vi "Pre Launch Init.vi"(11 "VMR Actor in":refnum<class "VMR Actor.lvclass">) -> (0 "error out":errorcluster, 3 "VMR Actor out":refnum<class "VMR Actor.lvclass">)   [LabVIEW 2022 SP3, in "VMR Server.lvlib" / "VMR Actor.lvclass"]
doc: "(<B>Filename</B>: Actor Framework.lvlib:Actor.lvclass:Pre Launch Init.vi)\n\nDefines behavior that occurs after the Launch Actor method is invoked but before the actor's Actor Core method begins running.\n\nThe Pre Launch Init method is guaranteed to finish before the Launch Actor method returns to its caller and before the actor itself receives any messages. Any references that the Pre Launch Init method obtains are guaranteed to have the same lifetime as the actor itself. Any errors that the Pre Launch Init method returns will abort the launch.\n\nBy default, this method does nothing. A descendant class may override it to define behavior."
uses:
  VMR Actor.lvclass
  <vilib>/ActorFramework/Actor/Actor.lvclass
  VMR Actor.lvclass/VMR Actor.ctl
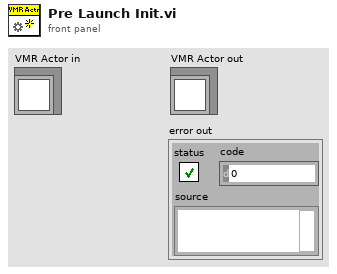
[diagram p1: front panel]
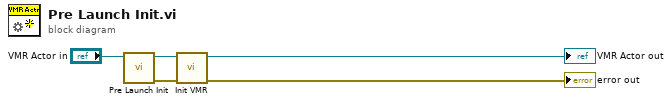
[diagram p0: block diagram]
diagram:
  n1 = call-parent "Pre Launch Init.vi"("Actor in"="VMR Actor in") -> ("error out"=w4:errorcluster, "Actor out"=w2:refnum<class "VMR Actor.lvclass">)  [unwired: 9 in]
  n2 = call "Init VMR.vi"("error in (no error)"=w4, "VMR Actor in"=w2) -> ("error out"=→"error out":errorcluster, "VMR Actor out"=→"VMR Actor out":refnum<class "VMR Actor.lvclass">)  [unwired: 8 in]
